vi "Queue Error Handler.vi"(8 "Error In":errorcluster) -> (0 "Error Out":errorcluster)   [LabVIEW 2013]
doc: "This sub-VI checks whether the error on an error bus is associated with a queue being disabled, and clears\nthe error if so."
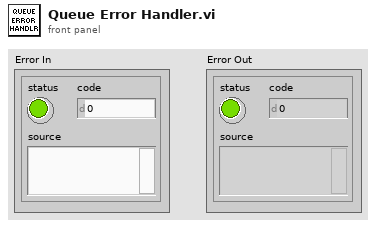
[diagram p1: front panel]
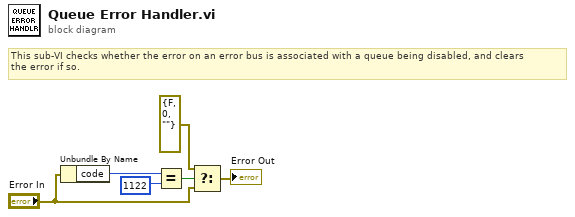
[diagram p0: block diagram]
diagram:
  # "This sub-VI checks whether the error on an error bus is associated with a queue being disabled, and clears\nthe error if so."
  n1 = Unbundle By Name("Error In") -> ("code"=w6:i32)
  n2 = Equal?(x=w6, y=1122) -> (x = y?=w4:bool)
  n3 = Select(t=errorcluster {"status"=FALSE, "code"=0, "source"=""}, s=w4, f="Error In") -> (s? t:f=→"Error Out":errorcluster)
